vi "MT Apply Matched Filter (CPM).vi"(0 "input complex waveform":T1={"t0"=0.0, "dt"=1.0, "Y"=[]} {"Y" format="%.3f"; "dt" format="%^.2e"; "t0" format="%.4f"}, 5 "matched filter coefficients":dbl[](array[numeric]) format="%^.2e", 7 "samples per symbol (16)":i32=16, 11 "error in (no error)":errorcluster, 13 "reset? (T)":bool=TRUE) -> (4 "output phase waveform":cluster{"t0":dbl, "dt":dbl, "Y":dbl[]} {"Y" min=0.0 max=127.0 format="%.3f"; "dt" format="%^.2e"; "t0" format="%.4f"}, 15 "error out":errorcluster)   [LabVIEW 2020, in "niDMT.lvlib"]
doc: "This polymorphic instance applies a matched filter to a specified CPM-modulated waveform. The VI first performs phase differentiation, followed by matched filtering on the phase of the input complex waveform."
uses:
  <vilib>/addons/Modulation/niDMT.lvlib
  <vilib>/addons/Modulation/Analog/controls/Complex Data Waveform.ctl
  <vilib>/addons/Modulation/niAMT.lvlib
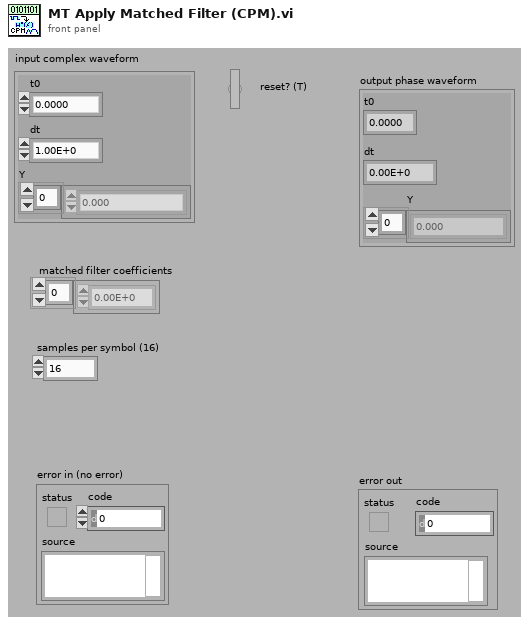
[diagram p1: front panel]
types:
  T1 = typedef "niAMT.lvlib/Complex Data Waveform.ctl" = cluster{"t0":dbl, "dt":dbl, "Y":cdb[]}
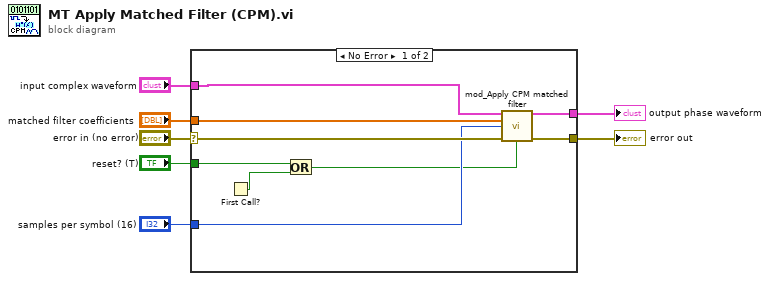
[diagram p0: block diagram]
diagram:
  n1 = case shown="No Error" "error in (no error)" {
    selector: "error in (no error)" -> [w13 w17]
    tunnel: "input complex waveform" -> [w11 _]
    tunnel: [w14 w17] -> w2
    tunnel: "matched filter coefficients" -> [w9 _]
    tunnel: "reset? (T)" -> [w16 _]
    tunnel: [w12 _] -> w3
    tunnel: "samples per symbol (16)" -> [w10 _]
    frame No Error {
      n2 = First Call?() -> (First Call?: T/F=w15:bool)
      n3 = Or(x=w16, y=w15) -> (x .or. y?=w8:bool)
      n4 = call <vilib>:"mod_Apply CPM matched filter.vi"("input complex waveform"=w11, "matched filter coefficients"=w9, "samples per symbol (16)"=w10, "error in (no error)"=w13, "reset? (T)"=w8) -> ("output phase waveform"=w12:cluster{"t0":dbl, "dt":dbl, "Y":dbl[]}, "error out"=w14:errorcluster)  [unwired: 1 in, 8 out]
    }
    frame Error {
    }
  }
  "output phase waveform" <- w3
  "error out" <- w2
